vi "Create-Delete Measurements.vi"(5 "Measurements":i32[](array[ring])=[0, 1, 2, 3] items=["S11", "S21", "S12", "S22", "A", "B", "R1", "R2", "A/B", "B/A"], 7 "Measurement Name":string, 8 "error out":errorcluster, 9 "Mode (0: Create)":u16(ring) items=["Create", "Delete", "Select", "Delete All"], 10 "Channel (1)":i32=1, 11 "VISA session":refnum<visa-resource-name>) -> (0 "Error Out":errorcluster, 3 "VISA Resource Name Out":refnum<visa-resource-name>)   [LabVIEW 2019, in "N5222A PNA.lvclass"]
doc: "Create multiple measurements\nCreate new traces in the same window (1)"
uses:
  N5222A PNA.lvclass
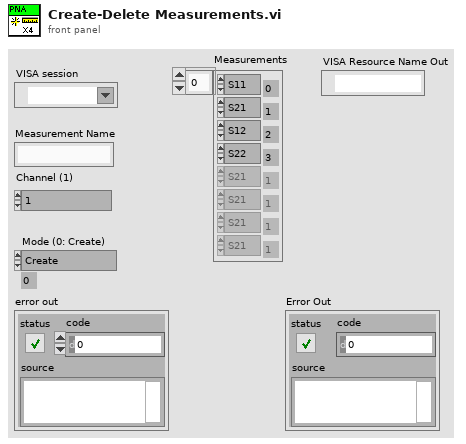
[diagram p1: front panel]
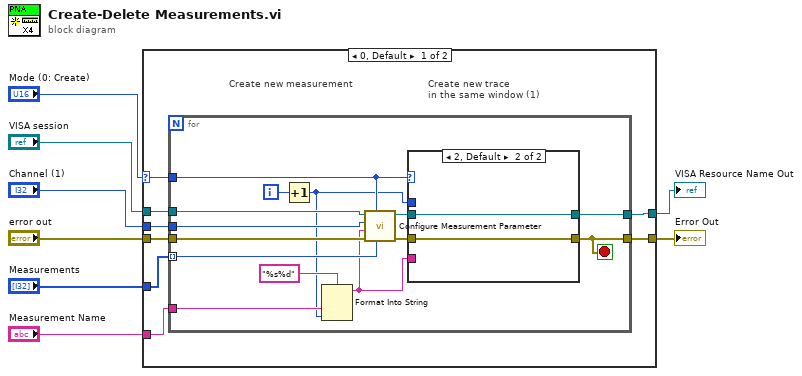
[diagram p0: block diagram]
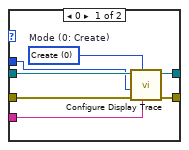
[diagram p2: hidden frame]
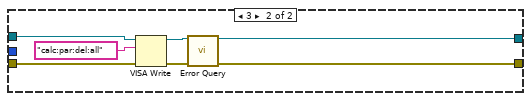
[diagram p3: hidden frame]
diagram:
  n1 = case shown="0, Default" "Mode (0: Create)" {
    selector: "Mode (0: Create)" -> [w9 _]
    tunnel: "VISA session" -> [w16 w41]
    tunnel: "Measurements" -> [w15 _]
    tunnel: "Measurement Name" -> [w14 _]
    tunnel: "Channel (1)" -> [w13 _]
    tunnel: [w12 w43] -> w4
    tunnel: [w11 w44] -> w3
    tunnel: "error out" -> [w10 w42]
    frame 0, Default {
      # "Create new trace\nin the same window (1)"
      # "Create new measurement"
      n2 = for {
        tunnel: w15 -> [w30] mode=indexing
        tunnel: w14 -> [w18]
        tunnel: w13 -> [w29]
        tunnel: w16 -> [w25]
        tunnel: [w24] -> w11
        tunnel: [w23] -> w12
        tunnel: w10 -> [w22]
        tunnel: w9 -> [w20]
        i -> [w26]
        stop <- w23 stop-if-true
        n3 = Increment(x=w26) -> (x+1=w17:i32)
        n4 = Format Into String(format string="%s%d", w18, w17) -> (resulting string=w21:string)  [unwired: 2 in, 1 out]
        n5 = call <instrlib>:"Configure Measurement Parameter.vi"("Measurement Type (0: S11)"=w30, "Mode (0: Create)"=w20, "Error In (no error)"=w22, "Measurement Name (MY_MEAS)"=w21, "Channel (1)"=w29, "VISA Resource Name"=w25) -> ("Error Out"=w27:errorcluster, "VISA Resource Name Out"=w28:refnum<visa-resource-name>)  [unwired: 4 in]
        n6 = case shown="2, Default" w20 {
          tunnel: w28 -> [w36 w39]
          tunnel: w27 -> [w35 w38]
          tunnel: [w34 w39] -> w24
          tunnel: [w33 w38] -> w23
          tunnel: w21 -> [w32 _]
          tunnel: w17 -> [w31 _]
          frame 0 {
            w37 = u16 0 items=["Create", "Delete"]  # Mode (0: Create)
            n7 = call <instrlib>:"Configure Display Trace.vi"("Measurement Name (MY_MEAS)"=w32, "Mode (0: Create)"=w37, "Error In (no error)"=w35, "Display Trace (1)"=w31, "VISA Resource Name"=w36) -> ("Error Out"=w33:errorcluster, "VISA Resource Name Out"=w34:refnum<visa-resource-name>)  [unwired: 5 in]
          }
          frame 2, Default {
          }
        }
      }
    }
    frame 3 {
      n8 = VISA Write(VISA resource name=w41, write buffer="calc:par:del:all", error in (no error)=w42) -> (VISA resource name out=w46:refnum<visa-resource-name>, error out=w45:errorcluster)  [unwired: 1 out]
      n9 = call <instrlib>:"Error Query.vi"("VISA Resource Name"=w46, "error in (no error)"=w45) -> ("VISA Resource Name Out"=w44:refnum<visa-resource-name>, "error out"=w43:errorcluster)  [unwired: 10 in, 2 out]
    }
  }
  "Error Out" <- w4
  "VISA Resource Name Out" <- w3
